vi "TempRampDoubleHeater.vi"(0 "IP Address Heater 1":string="192.168.12.200", 1 "Port Number Heater 1":u16=2000, 2 "IP Address Heater 2":string="192.168.12.201", 3 "Port Number Heater 2":u16=2000, 4 "Start T1 (C)":dbl=100.0, 5 "End T1 (C)":dbl=105.0, 6 "Duration of Ramp (min)":dbl=5.0, 7 "Additional Temperature for Heater 2":dbl=50.0, 8 "Temperature Log Interval (s)":dbl=5.0, 11 "Error In (no error)":errorcluster) -> (13 "Error Out":errorcluster, 14 "Heater 1 Temperature (C)":dbl=101.1 format="%.2f", 15 "Heater 2 Temperature (C)":dbl=153.3 format="%.2f", 16 "Setpoint 1 Diagnosis":string="W01", 17 "Setpoint 2 Diagnosis":string="W01", 18 "SP Heater 1":dbl=100.0 format="%.2f", 19 "SP Heater 2":dbl=150.0 format="%.2f")   [LabVIEW 2013, in "ovenCtrl.lvlib"]
uses:
  ovenCtrl.lvlib
panel:
  # "Inputs"
  # "Device Address"
  # "Temperature Ramp"
  # "Outputs"
  # "Diagnosis"
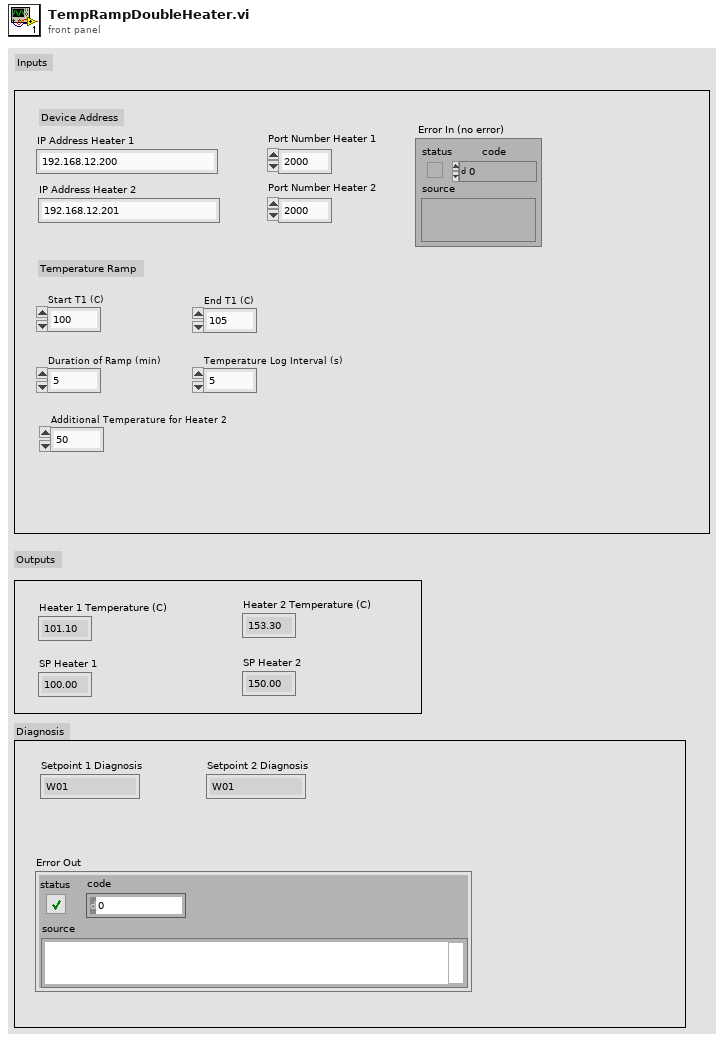
[diagram p1: front panel]
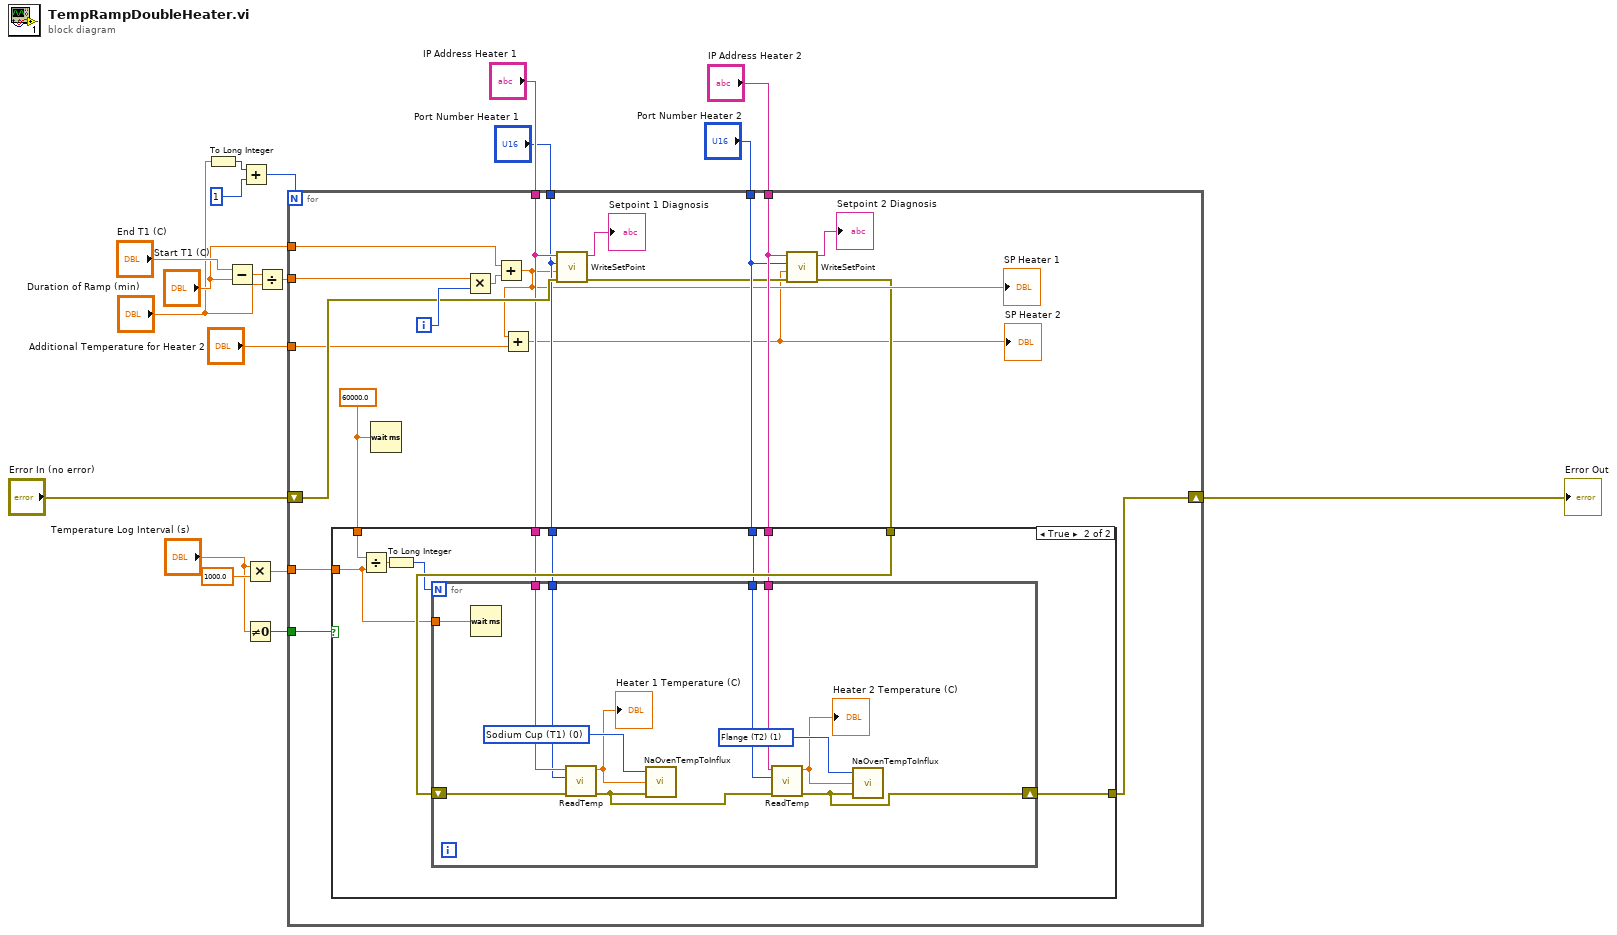
[diagram p0: block diagram]
diagram:
  n1 = To Long Integer(number="Duration of Ramp (min)") -> (32bit integer=w15:i32)
  n2 = Subtract(x="End T1 (C)", y="Start T1 (C)") -> (x-y=w18:dbl)
  n3 = Add(x=w15, y=1) -> (x+y=w13:i32)
  n4 = Multiply(x="Temperature Log Interval (s)", y=1000.0) -> (x*y=w3:dbl)
  n5 = Not Equal To 0?(x="Temperature Log Interval (s)") -> (x != 0?=w1:bool)
  n6 = Divide(x=w18, y="Duration of Ramp (min)") -> (x/y=w16:dbl)
  n7 = for {
    N: w13 -> [_]
    tunnel: "Start T1 (C)" -> [w39]
    tunnel: w16 -> [w36]
    tunnel: "IP Address Heater 1" -> [w30]
    tunnel: "Port Number Heater 1" -> [w29]
    shift-right: [w26] -> w6
    shift-left: "Error In (no error)" -> [w34]
    tunnel: "IP Address Heater 2" -> [w28]
    tunnel: "Port Number Heater 2" -> [w27]
    tunnel: "Additional Temperature for Heater 2" -> [w33]
    tunnel: w3 -> [w25]
    tunnel: w1 -> [w24]
    i -> [w38]
    w31 = 60000.0 ("y")
    n8 = Wait (ms)(milliseconds to wait=w31) -> ()  [unwired: 1 out]
    n9 = Multiply(x=w36, y=w38) -> (x*y=w37:dbl)
    n10 = Add(x=w39, y=w37) -> (x+y=w22:dbl)
    "SP Heater 1" <- w22
    n11 = Add(x=w22, y=w33) -> (x+y=w20:dbl)
    "SP Heater 2" <- w20
    n12 = call "WriteSetPoint.vi"("error in (no error)"=w34, "Setpoint (C)"=w22, "Port Number"=w29, "IP Address"=w30) -> ("error out"=w23:errorcluster, "Output Reading"=→"Setpoint 1 Diagnosis":string)  [unwired: 6 in]
    n13 = call "WriteSetPoint.vi"("error in (no error)"=w23, "Setpoint (C)"=w20, "Port Number"=w27, "IP Address"=w28) -> ("error out"=w21:errorcluster, "Output Reading"=→"Setpoint 2 Diagnosis":string)  [unwired: 6 in]
    n14 = case shown="True" w24 {
      tunnel: w31 -> [_ w50]
      tunnel: w21 -> [w40 w49]
      tunnel: w30 -> [_ w48]
      tunnel: w29 -> [_ w47]
      tunnel: w28 -> [_ w46]
      tunnel: w27 -> [_ w45]
      tunnel: [w40 w44] -> w26
      tunnel: w25 -> [_ w41]
      frame False {
      }
      frame True {
        n15 = Divide(x=w50, y=w41) -> (x/y=w43:dbl)
        n16 = To Long Integer(number=w43) -> (32bit integer=w42:i32)
        n17 = for {
          N: w42 -> [_]
          shift-right: [w51] -> w44
          shift-left: w49 -> [w57]
          tunnel: w48 -> [w62]
          tunnel: w47 -> [w61]
          tunnel: w46 -> [w60]
          tunnel: w45 -> [w59]
          tunnel: w41 -> [w58]
          w54 = u16 1 items=["Sodium Cup (T1)", "Flange (T2)"] ("Thermocouple")
          w56 = u16 0 items=["Sodium Cup (T1)", "Flange (T2)"] ("Thermocouple")
          n18 = Wait (ms)(milliseconds to wait=w58) -> ()  [unwired: 1 out]
          n19 = call "ReadTemp.vi"("error in (no error)"=w57, "Port Number"=w61, "IP Address"=w62) -> ("error out"=w52:errorcluster, "Temperature"=w55:dbl)  [unwired: 7 in]
          "Heater 1 Temperature (C)" <- w55
          n20 = call "NaOvenTempToInflux.vi"("error in (no error)"=w52, "Temperature Input"=w55, "Thermocouple"=w56) -> ()  [unwired: 1 in, 2 out]
          n21 = call "ReadTemp.vi"("error in (no error)"=w52, "Port Number"=w59, "IP Address"=w60) -> ("error out"=w51:errorcluster, "Temperature"=w53:dbl)  [unwired: 7 in]
          "Heater 2 Temperature (C)" <- w53
          n22 = call "NaOvenTempToInflux.vi"("error in (no error)"=w51, "Temperature Input"=w53, "Thermocouple"=w54) -> ()  [unwired: 1 in, 2 out]
        }
      }
    }
  }
  "Error Out" <- w6
